vi "test_psmc.vi"() -> ()   [LabVIEW 2014]
uses:
  <vilib>/ptbypt/NI_PtbyPt.lvlib
panel:
  in  "pd":dbl
  out "reference vs actual":T1(graph)={"M1 desired speed"=-0.04979126824650304, "M1 position"=nan}
  in  "stop":bool
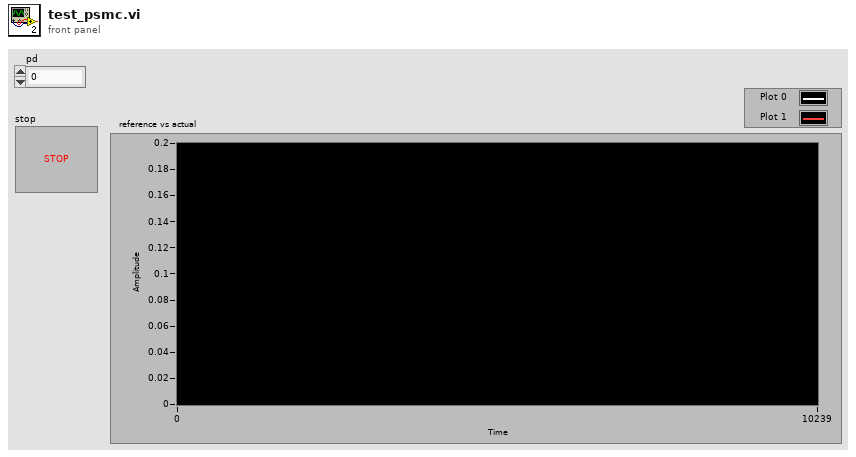
[diagram p1: front panel]
types:
  T1 = cluster{"M1 desired speed":dbl, "M1 position":dbl}
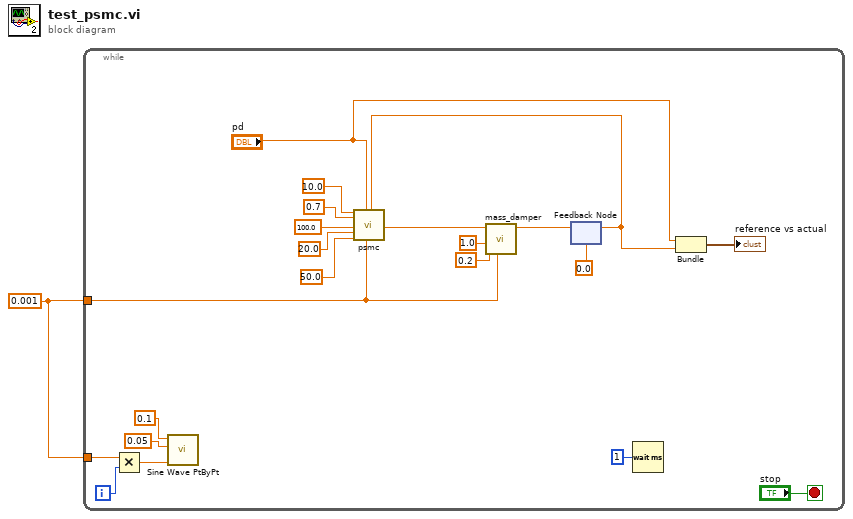
[diagram p0: block diagram]
diagram:
  w1 = 0.001 ("T")
  n1 = while {
    tunnel: w1 -> [w17]
    tunnel: w1 -> [w3]
    i -> [w18]
    stop <- "stop" stop-if-true
    n2 = Multiply(x=w17, y=w18) -> (x*y=w21:dbl)
    n3 = call <vilib>:"Sine Wave PtByPt.vi"("time"=w21, "frequency"=0.05, "amplitude"=0.1) -> ()  [unwired: 1 in, 1 out]
    n4 = feedback #1(0.0 ("integral x(t)")) -> (w11:dbl)
    n5 = call "psmc.vi"("F"=10.0, "H"=0.7, "K"=100.0, "L"=20.0, "B"=50.0, "pd"="pd", "T"=w3, "p"=w11) -> ("f"=w7:dbl)  [unwired: 11 in]
    n6 = call "mass_damper.vi"("dt"=w3, "B"=0.2, "Mass"=1.0, "f(t)"=w7) -> ("x(t)"=w6:dbl)  [unwired: 5 in, 2 out]
    n7 = feedback-in #1(w6) -> ()
    n8 = Wait (ms)(milliseconds to wait=u32 1) -> ()  [unwired: 1 out]
    n9 = Bundle("pd"="pd", "integral x(t)"=w11) -> (→"reference vs actual":cluster{"pd":dbl, "integral x(t)":dbl})  [unwired: 1 in]
  }
